vi "Host_HoppingScan(XZCurrEnhanced).vi"() -> ()   [LabVIEW 2014]
uses:
  <vilib>/userdefined/High Color/nirio_resource_hc.ctl
  <vilib>/Native 3D Graph/xcontrol/3DPC_SurfacePlot.xctl
  <vilib>/Instr/_visa.llb/VISA Configure Serial Port (Instr).vi
  <vilib>/FPGAPlugInAG/PCIe-7851R/niLvFpga_Open_PCIe-7851R.vi
  <vilib>/rvi/interface/common/dynamic/niFpgaDynamicAddResources.vi
  <vilib>/Utility/error.llb/Error Cluster From Error Code.vi
  <vilib>/rvi/errors/niLvFpgaAdjustHostInterfaceError.vi
  <vilib>/FPGAPlugInAG/Dynamic/niLvFpga_Close_Dynamic.vi
  <vilib>/rvi/interface/nirviOpenFPGA/nirviOpenFPGA.xnode
  FPGA Bitfiles/XZFPGAWithinHopp_FPGATarget_HoppingStep(Nonl_SD+4nnFSMrs.lvbitx
  <vilib>/rvi/interface/nirviReadWriteControl/nirviReadWriteControl.xnode
  <vilib>/rvi/interface/nirviMethod/nirviMethod.xnode
  <vilib>/rvi/interface/nirviCloseFPGA/nirviCloseFPGA.xnode
  NiFpgaLv.dll
  <vilib>/rvi/interface/Simulation/niFpgaSimulationCallBeginRW.vi
  <vilib>/FPGAPlugInAG/Dynamic/niLvFpga_ReadFifo_Dynamic.vi
  <vilib>/rvi/errors/niLvFpgaMergeErrorWithErrorCode.vi
  <vilib>/FPGAPlugInAG/Dynamic/niLvFpga_StopFifo_Dynamic.vi
panel:
  in  "FluctuationLimitRange":i32
  in  "CheckNum":i32
  out "XGetNum":u32
  in  "BottomSleep us":i32
  in  "UpperSleep us":i32
  out "SecElapsed s":dbl
  in  "UseCompensation":bool
  in  "Compensation / line":i32
  in  "RelativeWithdraw index":i32
  out "YPresPos":i32
  out "XBuffer":u32
  out "Waveform Chart":i32(graph)
  out "3D Graph":refnum<class "Base Datatype.lvclass">[](xcontrol)
  in  "stop":bool
  in  "ZOffset index":i32
  out "YPos?":dbl
  in  "YNum":i16
  in  "XNum":i16
  in  "YStepLen um":dbl format="%#_13g"
  in  "XStepMultiplier / 1.5nm":i16
  in  "XInitPos um":dbl format="%#_13g"
  in  "YInitPos um":dbl format="%#_13g"
  in  "PIXZ":T1
  out "ERR?":string
  in  "PIYDigital":refnum<visa-resource-name>
  # "Note: \nCheckNum用来设置扫描次数，不填的话，默认10次确认\n（建议不要低于10次）\nFluctuationLimitRange设置探针在Z方向允许的波动距离限制index，\n若上下任意超过该index，则进行CheckNum的单点确认次数"
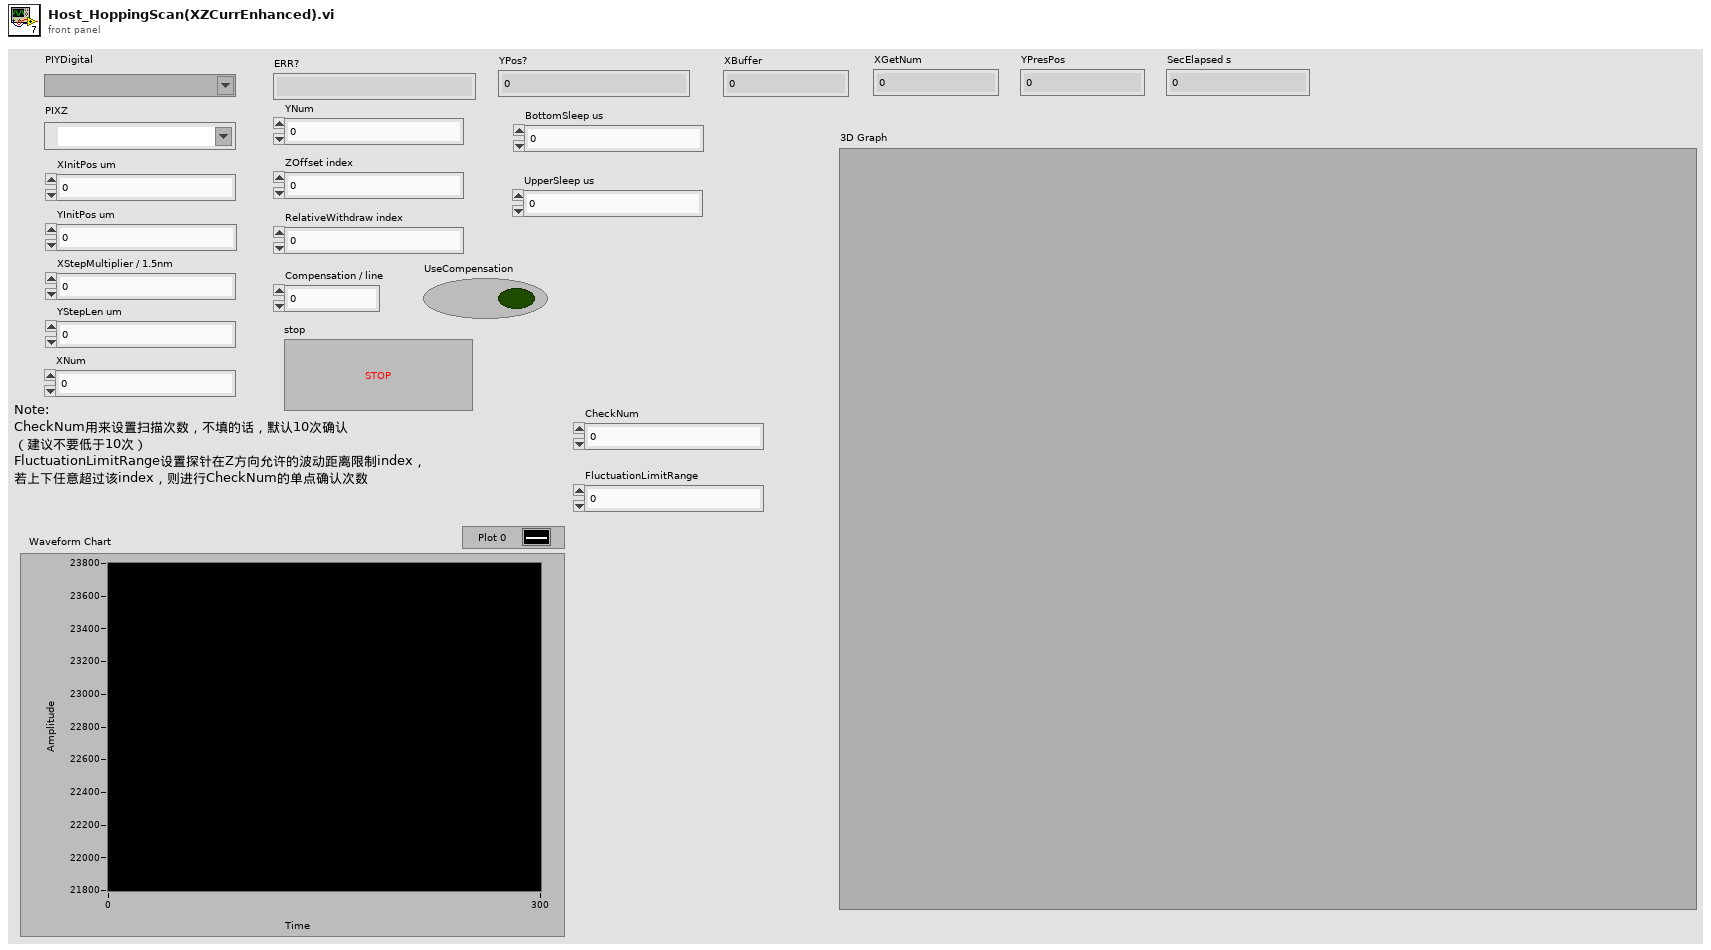
[diagram p1: front panel]
types:
  T1 = typedef "nirio_resource_hc.ctl" = tag
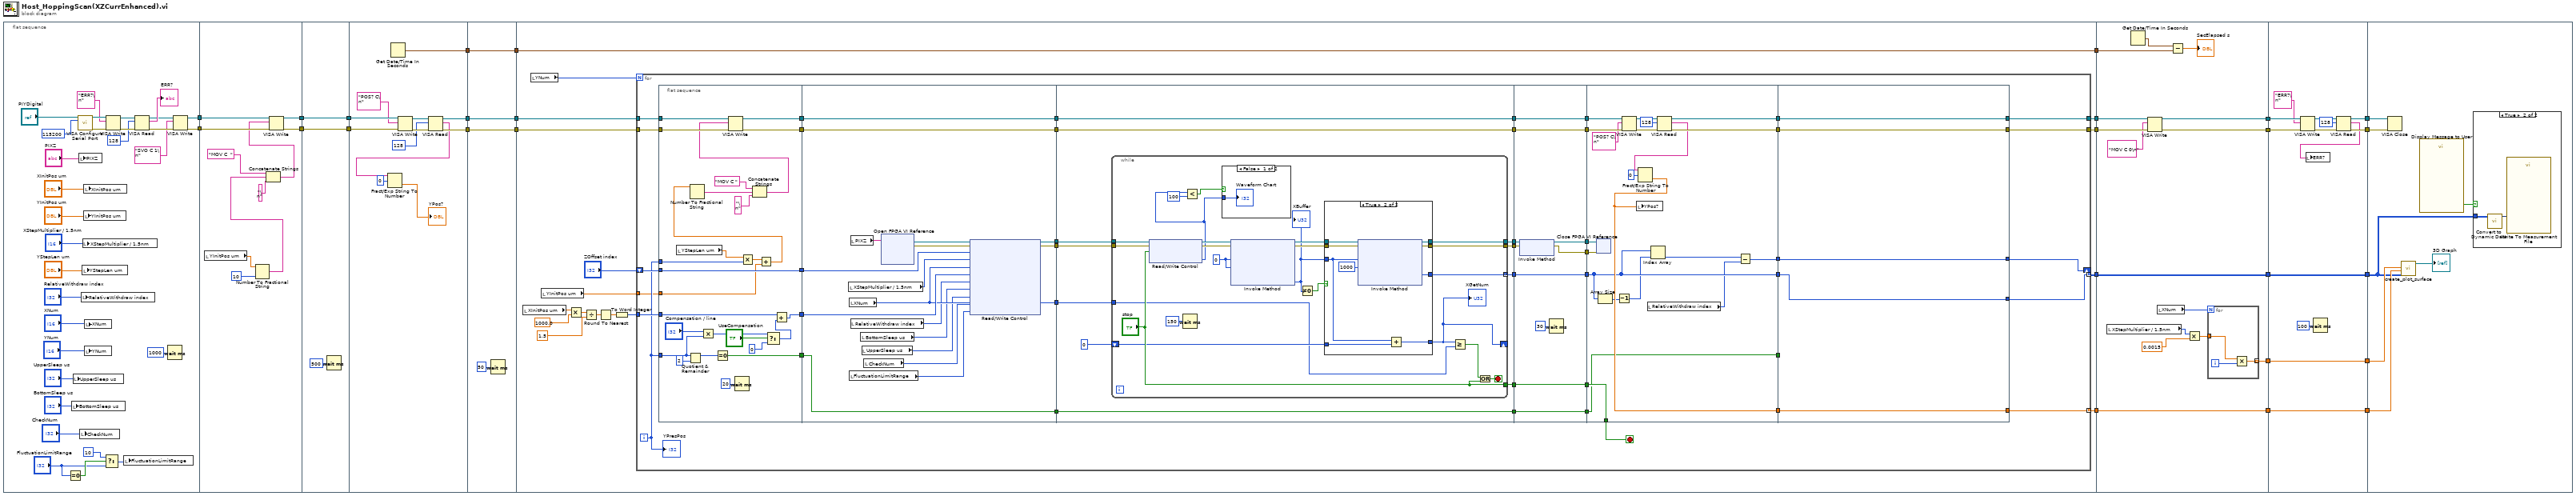
[diagram p0: block diagram]
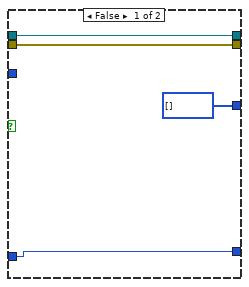
[diagram p3: hidden frame]
diagram:
  n1 = flat-sequence {
    tunnel: [w37] -> w27
    tunnel: [w36] -> w26
    tunnel: w27 -> [w67]
    tunnel: w26 -> [w66]
    tunnel: [w62] -> w25
    tunnel: [w61] -> w24
    tunnel: w25 -> [w69]
    tunnel: w24 -> [w68]
    tunnel: [w69] -> w23
    tunnel: [w68] -> w22
    tunnel: w23 -> [w82]
    tunnel: w22 -> [w81]
    tunnel: [w76] -> w21
    tunnel: [w75] -> w20
    tunnel: [w71] -> w2
    tunnel: w21 -> [w85]
    tunnel: w20 -> [w84]
    tunnel: [w85] -> w19
    tunnel: [w84] -> w18
    tunnel: [w83] -> w3
    tunnel: w2 -> [w83]
    tunnel: w19 -> [w102]
    tunnel: w18 -> [w101]
    tunnel: [w93] -> w17
    tunnel: [w92] -> w16
    tunnel: [w91] -> w11
    tunnel: [w90] -> w10
    tunnel: w3 -> [w87]
    tunnel: [w87] -> w1
    tunnel: w17 -> [w287]
    tunnel: w16 -> [w286]
    tunnel: [w284] -> w15
    tunnel: [w283] -> w14
    tunnel: w11 -> [w276]
    tunnel: w10 -> [w277]
    tunnel: [w278] -> w9
    tunnel: [w277] -> w6
    tunnel: [w276] -> w4
    tunnel: w1 -> [w275]
    tunnel: w15 -> [w303]
    tunnel: w14 -> [w302]
    tunnel: [w297] -> w13
    tunnel: [w296] -> w12
    tunnel: w9 -> [w293]
    tunnel: [w293] -> w8
    tunnel: [w292] -> w7
    tunnel: w6 -> [w292]
    tunnel: [w291] -> w5
    tunnel: w4 -> [w291]
    tunnel: w13 -> [w310]
    tunnel: w12 -> [w309]
    tunnel: w8 -> [w307]
    tunnel: w7 -> [w306]
    tunnel: w5 -> [w304]
    frame #0 {
      n2 = Equal To 0?(x="FluctuationLimitRange") -> (x = 0?=w31:bool)
      n3 = local write "BottomSleep us"("BottomSleep us") -> ()
      n4 = local write "UpperSleep us"("UpperSleep us") -> ()
      n5 = call-poly "VISA Configure Serial Port"("VISA resource name"="PIYDigital", "baud rate (9600)"=u32 115200) -> ("VISA resource name out"=w55:refnum<visa-resource-name>, "error out"=w54:errorcluster)  [unwired: 12 in]
      n6 = local write "PIXZ"("PIXZ") -> ()
      n7 = local write "CheckNum"("CheckNum") -> ()
      n8 = local write "RelativeWithdraw index"("RelativeWithdraw index") -> ()
      n9 = local write "YStepLen um"("YStepLen um") -> ()
      n10 = local write "XStepMultiplier / 1.5nm"("XStepMultiplier / 1.5nm") -> ()
      n11 = local write "YInitPos um"("YInitPos um") -> ()
      n12 = local write "XInitPos um"("XInitPos um") -> ()
      n13 = local write "XNum"("XNum") -> ()
      n14 = local write "YNum"("YNum") -> ()
      n15 = Select(t=10, s=w31, f="FluctuationLimitRange") -> (s? t:f=w28:i32)
      n16 = VISA Write(VISA resource name=w55, write buffer="ERR?\n", error in (no error)=w54) -> (VISA resource name out=w52:refnum<visa-resource-name>, error out=w51:errorcluster)  [unwired: 1 out]
      n17 = local write "FluctuationLimitRange"(w28) -> ()
      n18 = VISA Read(VISA resource name=w52, byte count=u32 128, error in (no error)=w51) -> (VISA resource name out=w39:refnum<visa-resource-name>, read buffer=→"ERR?":string, error out=w38:errorcluster)  [unwired: 1 out]
      n19 = Wait (ms)(milliseconds to wait=u32 1000) -> ()  [unwired: 1 out]
      n20 = VISA Write(VISA resource name=w39, write buffer="SVO C 1\n", error in (no error)=w38) -> (VISA resource name out=w37:refnum<visa-resource-name>, error out=w36:errorcluster)  [unwired: 1 out]
    }
    frame #1 {
      n21 = local read "YInitPos um"() -> (w60:dbl)
      n22 = Number To Fractional String(number=w60, precision (6)=i16 10) -> (F-format string=w58:string)  [unwired: 2 in]
      n23 = Concatenate Strings("MOV C  " ("write buffer"), w58, "\n" ("string")) -> (w63:string)
      n24 = VISA Write(VISA resource name=w67, write buffer=w63, error in (no error)=w66) -> (VISA resource name out=w62:refnum<visa-resource-name>, error out=w61:errorcluster)  [unwired: 1 out]
    }
    frame #2 {
      n25 = Wait (ms)(milliseconds to wait=u32 500) -> ()  [unwired: 1 out]
    }
    frame #3 {
      n26 = Get Date/Time In Seconds() -> (seconds since 1Jan1904=w71:timestamp)
      n27 = VISA Write(VISA resource name=w82, write buffer="POS? C\n", error in (no error)=w81) -> (VISA resource name out=w79:refnum<visa-resource-name>, error out=w78:errorcluster)  [unwired: 1 out]
      n28 = VISA Read(VISA resource name=w79, byte count=u32 128, error in (no error)=w78) -> (VISA resource name out=w76:refnum<visa-resource-name>, read buffer=w74:string, error out=w75:errorcluster)  [unwired: 1 out]
      n29 = Fract/Exp String To Number(string=w74, offset=0) -> (number=→"YPos?":dbl)  [unwired: 2 in, 1 out]
    }
    frame #4 {
      n30 = Wait (ms)(milliseconds to wait=u32 50) -> ()  [unwired: 1 out]
    }
    frame #5 {
      n31 = local read "XInitPos um"() -> (w95:dbl)
      n32 = local read "YNum"() -> (w103:i16)
      n33 = local read "YInitPos um"() -> (w88:dbl)
      n34 = Multiply(x=w95, y=1000.0) -> (x*y=w97:dbl)
      n35 = Divide(x=w97, y=1.5) -> (x/y=w99:dbl)
      n36 = Round To Nearest(number=w99) -> (nearest integer value=w100:dbl)
      n37 = To Word Integer(number=w100) -> (16bit integer=w94:i16)
      n38 = for {
        N: w103 -> [_]
        tunnel: w102 -> [w146]
        tunnel: w101 -> [w145]
        tunnel: w94 -> [w139]
        tunnel: [w131] -> w93
        tunnel: [w130] -> w92
        tunnel: [w111] -> w91 mode=indexing
        tunnel: [w122] -> w90 mode=indexing
        shift-right: [w117] -> _
        shift-left: "ZOffset index" -> [w120]
        tunnel: w88 -> [w104]
        i -> [w119]
        stop <- w125 stop-if-true
        n39 = flat-sequence {
          tunnel: w146 -> [w171]
          tunnel: w145 -> [w170]
          tunnel: w119 -> [w172]
          tunnel: [w169] -> w144
          tunnel: [w168] -> w143
          tunnel: [w153] -> w140
          tunnel: w139 -> [w154]
          tunnel: [w162] -> w121
          tunnel: w120 -> [w162]
          tunnel: w119 -> [w151]
          tunnel: [w159] -> w118
          tunnel: w104 -> [w156]
          tunnel: [w186] -> w142
          tunnel: [w185] -> w141
          tunnel: [w181] -> w138
          tunnel: [w180] -> w137
          tunnel: [w182] -> w134
          tunnel: w121 -> [w179]
          tunnel: w140 -> [w183]
          tunnel: w143 -> [w185]
          tunnel: w144 -> [w186]
          tunnel: w118 -> [w178]
          tunnel: [w178] -> w110
          tunnel: w142 -> [w200]
          tunnel: w141 -> [w199]
          tunnel: w138 -> [w192]
          tunnel: w137 -> [w191]
          tunnel: [w200] -> w136
          tunnel: [w199] -> w135
          tunnel: w134 -> [w198]
          tunnel: [w197] -> w133
          tunnel: [w196] -> w132
          tunnel: [w195] -> w127
          tunnel: [w194] -> w123
          tunnel: w110 -> [w193]
          tunnel: [w193] -> w109
          tunnel: w136 -> [w246]
          tunnel: w135 -> [w245]
          tunnel: w133 -> [w241]
          tunnel: w132 -> [w240]
          tunnel: [w246] -> w129
          tunnel: [w245] -> w128
          tunnel: w127 -> [w243]
          tunnel: [w243] -> w126
          tunnel: [w242] -> w124
          tunnel: w123 -> [w242]
          tunnel: w109 -> [w239]
          tunnel: [w239] -> w108
          tunnel: [w238] -> w106
          tunnel: [w237] -> w105
          tunnel: w129 -> [w267]
          tunnel: w128 -> [w266]
          tunnel: w126 -> [w257]
          tunnel: [w257] -> w125
          tunnel: w124 -> [w254]
          tunnel: [w263] -> w116
          tunnel: [w262] -> w115
          tunnel: [w254] -> w114
          tunnel: [w256] -> w113
          tunnel: [w250] -> w112
          tunnel: w108 -> [w249]
          tunnel: [w249] -> w107
          tunnel: w106 -> [w248]
          tunnel: w105 -> [w247]
          tunnel: [w269] -> w117
          tunnel: [w270] -> w122
          tunnel: [w271] -> w130
          tunnel: [w272] -> w131
          tunnel: w116 -> [w272]
          tunnel: w115 -> [w271]
          tunnel: w114 -> [w268]
          tunnel: w113 -> [w270]
          tunnel: w112 -> [w269]
          tunnel: [w268] -> w111
          tunnel: w107 -> [_]
          frame #0 {
            n40 = local read "YStepLen um"() -> (w167:dbl)
            n41 = Quotient & Remainder(x=w151, y=2) -> (x-y*floor(x/y)=w160:i32)  [unwired: 1 out]
            n42 = Multiply(x="Compensation / line", y=w151) -> (x*y=w150:i32)
            n43 = Equal To 0?(x=w160) -> (x = 0?=w159:bool)
            n44 = Wait (ms)(milliseconds to wait=u32 20) -> ()  [unwired: 1 out]
            n45 = Multiply(x=w167, y=w172) -> (x*y=w157:dbl)
            n46 = Add(x=w157, y=w156) -> (x+y=w155:dbl)
            n47 = Number To Fractional String(number=w155) -> (F-format string=w166:string)  [unwired: 3 in]
            n48 = Concatenate Strings("MOV C " ("string"), w166, "\n" ("string")) -> (w163:string)
            n49 = VISA Write(VISA resource name=w171, write buffer=w163, error in (no error)=w170) -> (VISA resource name out=w169:refnum<visa-resource-name>, error out=w168:errorcluster)  [unwired: 1 out]
            n50 = Select(t=w150, s="UseCompensation", f=0) -> (s? t:f=w147:i32)
            n51 = Add(x=w154, y=w147) -> (x+y=w153:i32)
          }
          frame #1 {
            n52 = local read "XStepMultiplier / 1.5nm"() -> (w184:i16)
            n53 = local read "XNum"() -> (w182:i16)
            n54 = local read "FluctuationLimitRange"() -> (w173:i32)
            n55 = local read "PIXZ"() -> (w189:T1)
            n56 = local read "RelativeWithdraw index"() -> (w177:i32)
            n57 = local read "BottomSleep us"() -> (w176:i32)
            n58 = local read "UpperSleep us"() -> (w175:i32)
            n59 = local read "CheckNum"() -> (w174:i32)
            n60 = xnode "Open FPGA VI Reference"("resource name"=w189) -> ("FPGA VI Reference Out"=w188:refnum<k20>, "error out"=w187:errorcluster)  [unwired: 1 in]
            n61 = xnode "Read/Write Control"("FPGA VI Reference In"=w188, "error in"=w187, "ZOffset"=w179, "XStepIndex"=w184, "XNum"=w182, "XOffset"=w183, "RelativeWithdraw"=w177, "BottomSleep us"=w176, "UpperSleep us"=w175, "CheckNum"=w174, "ZLimitFluctuationRange"=w173) -> ("FPGA VI Reference Out"=w181:refnum<k20>, "error out"=w180:errorcluster)
          }
          frame #2 {
            n62 = while {
              tunnel: w192 -> [w215]
              tunnel: w191 -> [w214]
              tunnel: w198 -> [w202]
              tunnel: [w218] -> w197
              tunnel: [w217] -> w196
              tunnel: ["stop"] -> w195
              tunnel: [w211] -> w194 mode=concatenating
              shift-right: [w201] -> _
              shift-left: 0 -> [w204]
              stop <- w216 stop-if-true
              w221 = u32 0 ("Number of Elements")
              n63 = xnode "Read/Write Control"("FPGA VI Reference In"=w215, "error in"=w214, "stop"="stop") -> ("FPGA VI Reference Out"=w213:refnum<k20>, "error out"=w212:errorcluster, "Waveform Chart"=w207:i32)
              n64 = Wait (ms)(milliseconds to wait=u32 150) -> ()  [unwired: 1 out]
              n65 = Less?(x=w207, y=100) -> (x < y?=w208:bool)
              n66 = case shown="False" w208 {
                tunnel: w207 -> [w223 _]
                frame False {
                  "Waveform Chart" <- w223
                }
                frame True {
                }
              }
              n67 = xnode "Invoke Method"("FPGA VI Reference In"=w213, "error in"=w212, "Number of Elements"=w221, "Timeout (ms)"=w221) -> ("FPGA VI Reference Out"=w220:refnum<k20>, "error out"=w219:errorcluster, "Elements Remaining"=w205:u32)  [unwired: 1 out]
              "XBuffer" <- w205
              n68 = Not Equal To 0?(x=w205) -> (x != 0?=w206:bool)
              n69 = case shown="True" w206 {
                tunnel: w220 -> [w227 w236]
                tunnel: w219 -> [w226 w235]
                tunnel: [w227 w233] -> w218
                tunnel: [w226 w232] -> w217
                tunnel: [i16[] [] ("Data") w231] -> w211
                tunnel: w205 -> [_ w229]
                tunnel: w204 -> [w224 w230]
                tunnel: [w224 w228] -> w201
                frame False {
                }
                frame True {
                  n70 = xnode "Invoke Method"("FPGA VI Reference In"=w236, "error in"=w235, "Number of Elements"=w229, "Timeout (ms)"=1000) -> ("FPGA VI Reference Out"=w233:refnum<k20>, "error out"=w232:errorcluster, "Data"=w231:i16[])  [unwired: 1 out]
                  n71 = Add(x=w229, y=w230) -> (x+y=w228:u32)
                }
              }
              "XGetNum" <- w201
              n72 = Greater Or Equal?(x=w201, y=w202) -> (x >= y?=w203:bool)
              n73 = Or(x=w203, y="stop") -> (x .or. y?=w216:bool)
            }
          }
          frame #3 {
            n74 = xnode "Invoke Method"("FPGA VI Reference In"=w241, "error in"=w240) -> ("FPGA VI Reference Out"=w238:refnum<k20>, "error out"=w237:errorcluster)
            n75 = Wait (ms)(milliseconds to wait=u32 30) -> ()  [unwired: 1 out]
          }
          frame #4 {
            n76 = xnode "Close FPGA VI Reference"("FPGA VI Reference In"=w248, "error in"=w247) -> ()  [unwired: 1 out]
            n77 = Array Size(array=w254) -> (size(s)=w255:i32)
            n78 = Decrement(x=w255) -> (x-1=w253:i32)
            n79 = VISA Write(VISA resource name=w267, write buffer="POS? C\n", error in (no error)=w266) -> (VISA resource name out=w265:refnum<visa-resource-name>, error out=w264:errorcluster)  [unwired: 1 out]
            n80 = local read "RelativeWithdraw index"() -> (w251:i32)
            n81 = Index Array(array=w254, index=w253) -> (element=w252:i16)
            n82 = VISA Read(VISA resource name=w265, byte count=u32 128, error in (no error)=w264) -> (VISA resource name out=w263:refnum<visa-resource-name>, read buffer=w259:string, error out=w262:errorcluster)  [unwired: 1 out]
            n83 = Fract/Exp String To Number(string=w259, offset=0) -> (number=w256:dbl)  [unwired: 2 in, 1 out]
            n84 = local write "YPos?"(w256) -> ()
            n85 = Subtract(x=w252, y=w251) -> (x-y=w250:i32)
          }
          frame #5 {
          }
        }
        "YPresPos" <- w119
      }
    }
    frame #6 {
      n86 = local read "XStepMultiplier / 1.5nm"() -> (w281:i16)
      n87 = Get Date/Time In Seconds() -> (seconds since 1Jan1904=w274:timestamp)
      n88 = VISA Write(VISA resource name=w287, write buffer="MOV C 0\n", error in (no error)=w286) -> (VISA resource name out=w284:refnum<visa-resource-name>, error out=w283:errorcluster)  [unwired: 1 out]
      n89 = local read "XNum"() -> (w282:i16)
      n90 = Subtract(x=w274, y=w275) -> (x-y=→"SecElapsed s":dbl)
      n91 = Multiply(x=w281, y=0.0015) -> (x*y=w279:dbl)
      n92 = for {
        N: w282 -> [_]
        tunnel: w279 -> [w290]
        tunnel: [w288] -> w278 mode=indexing
        i -> [w289]
        n93 = Multiply(x=w290, y=w289) -> (x*y=w288:dbl)
      }
    }
    frame #7 {
      n94 = VISA Write(VISA resource name=w303, write buffer="ERR?\n", error in (no error)=w302) -> (VISA resource name out=w300:refnum<visa-resource-name>, error out=w299:errorcluster)  [unwired: 1 out]
      n95 = Wait (ms)(milliseconds to wait=u32 100) -> ()  [unwired: 1 out]
      n96 = VISA Read(VISA resource name=w300, byte count=u32 128, error in (no error)=w299) -> (VISA resource name out=w297:refnum<visa-resource-name>, read buffer=w295:string, error out=w296:errorcluster)  [unwired: 1 out]
      n97 = local write "ERR?"(w295) -> ()
    }
    frame #8 {
      n98 = VISA Close(VISA resource name=w310, error in (no error)=w309) -> ()  [unwired: 1 out]
      n99 = call <vilib>:"create_plot_surface.vi"("z matrix"=w304, "y vector"=w306, "x vector"=w307) -> ("plots out"=→"3D Graph":refnum<class "Base Datatype.lvclass">[])  [unwired: 2 in, 6 out]
      n100 = call "Display Message to User"() -> ("OK"=w305:bool)  [unwired: 10 in, 1 out]
      n101 = case shown="True" w305 {
        tunnel: w304 -> [_ w312]
        frame False {
        }
        frame True {
          n102 = call "Convert to Dynamic Data"("2D Array"=w312) -> ("Dynamic Data Type"=w311:dynamicdata)  [unwired: 3 in]
          n103 = call "Write To Measurement File"("Signals"=w311) -> ()  [unwired: 16 in, 3 out]
        }
      }
    }
  }
